vi "Read IPS PSU1 Current Voltage.vi"(8 "error in (no error)":errorcluster, 11 "Instrument.Oxford1820 in":refnum<class "Instrument.Oxford1820.lvclass">) -> (0 "error out":errorcluster, 1 "Voltage (V)":dbl, 2 "Current (A)":dbl, 3 "Instrument.Oxford1820 out":refnum<class "Instrument.Oxford1820.lvclass">)   [LabVIEW 2016, in "Instrument.Oxford1820.lvclass"]
uses:
  Instrument.Oxford1820.lvclass
  Instrument.Oxford1820.lvclass/Instrument.Oxford1820.ctl
  <instrlib>/Mercury iXX/Public/Libraries/Magnet/Open/Open Magnet Device.vi
  <instrlib>/Mercury iXX/Public/Libraries/Magnet/Signals/Read/Current (Read).vi
  <instrlib>/Mercury iXX/Public/Libraries/Magnet/Signals/Read/Voltage (Read).vi
  <instrlib>/Mercury iXX/Mercury iXX.lvlib
  <instrlib>/Mercury iXX/Public/Libraries/Magnet.lvlib
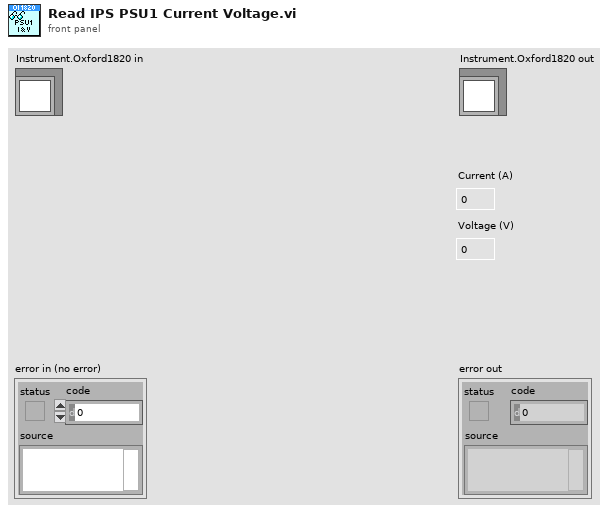
[diagram p1: front panel]
types:
  T1 = typedef "Mercury iXX.lvlib/Mercury Reference.ctl" = cluster{"Comms":refnum<visa-resource-name>, "Device ID":string[], "Comms Layer":T2, "Command":string, "Query reference":T3}
  T2 = typedef "Mercury iXX.lvlib/Comms Transport Layer.ctl" = enum16{"Ethernet TCP/IP", "USB", "ISOBus - RS-232", "GPIB"}
  T3 = typedef "Mercury iXX.lvlib/Query Dynamic Reference.ctl" = refnum<vi>
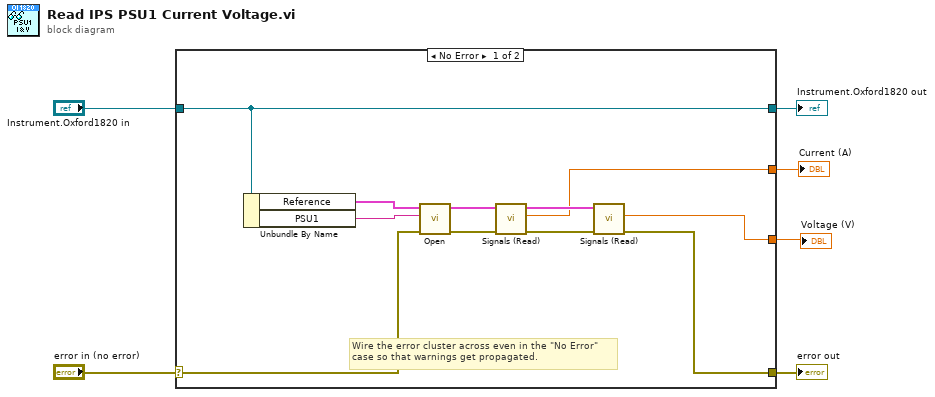
[diagram p0: block diagram]
diagram:
  n1 = case shown="No Error" "error in (no error)" {
    selector: "error in (no error)" -> [w12 w19]
    tunnel: [w7 w19] -> w5
    tunnel: [w15 w18] -> w3
    tunnel: "Instrument.Oxford1820 in" -> [w15 w18]
    tunnel: [w8 _] -> w2
    tunnel: [w9 _] -> w1
    frame No Error {
      # "Wire the error cluster across even in the \"No Error\"\ncase so that warnings get propagated."
      n2 = Unbundle By Name(w15) -> ("Reference"=w13:T1, "PSU1"=w14:string)
      n3 = call-poly <instrlib>:"Open.vi"("error in (no error)"=w12, "Device Identifier"=w14, "Mercury Reference In"=w13) -> ("error out"=w17:errorcluster, "Mercury Reference Out"=w16:T1)  [unwired: 7 out]
      n4 = call-poly <instrlib>:"Signals (Read).vi"("error in"=w17, "Mercury Reference In"=w16) -> ("error out"=w11:errorcluster, "Current"=w8:dbl, "Mercury Reference Out"=w10:T1)  [unwired: 1 in, 6 out]
      n5 = call-poly <instrlib>:"Signals (Read).vi"("error in"=w11, "Mercury Reference In"=w10) -> ("error out"=w7:errorcluster, "Voltage"=w9:dbl)  [unwired: 1 in, 7 out]
    }
    frame Error {
    }
  }
  "error out" <- w5
  "Instrument.Oxford1820 out" <- w3
  "Current (A)" <- w2
  "Voltage (V)" <- w1
